vi "Lab Environment Query.vi"() -> ()   [LabVIEW 2012]
uses:
  <vilib>/Utility/miscctls.llb/LVPointTypeDef.ctl
  <vilib>/addons/database/Auxilliary.llb/DB Tools Cursor Type.ctl
  <userlib>/_OpenG.lib/array/array.llb/Index 1D Array Elements (String)__ogtk.vi
  <vilib>/addons/database/Connection.llb/Conn Execute.vi
  <vilib>/addons/database/Recordset.llb/Rec Fetch Recordset Data (R).vi
  <vilib>/addons/database/Recordset.llb/Rec Destroy - Connection.vi
  <vilib>/Utility/file.llb/Write To Spreadsheet File (string).vi
  <vilib>/addons/database/_DB Variant To Data/Database Variant To Data.xnode
  <vilib>/addons/database/NI_Database_API.lvlib
panel:
  in  "stop":bool
  in  "Tab Control":T1(tab)
  in  "Active Y Scale":u16(ring) items=["Temperature (F)", "Pressure (torr)"]
  in  "X Maximum":dbl format="%<%I:%M:%S %p\n%m/%d/%Y>T"
  in  "X Autoscale":bool=TRUE
  in  "X Minimum":dbl format="%<%I:%M:%S %p\n%m/%d/%Y>T"
  in  "Y Autoscale":bool=TRUE
  in  "Y Maximum":dbl
  in  "Y Minimum":dbl
  in  "Plot":bool
  in  "Limits":T2
  in  "Lab Properties":i32[](listbox)
  out "XY Graph":cluster{ext[], dbl[]}[](graph)
  in  "Write":bool
  in  "Pull Data":bool
  in  "Limits 2":T2
  out "Lab Environment Data":string[][](table)
  in  "Save Path":path=path "C:/Users/Clavius/Desktop/Database Query files/New_Pelletron_Query.csv"
  out "error out":errorcluster
  in  "Clear Errors?":bool
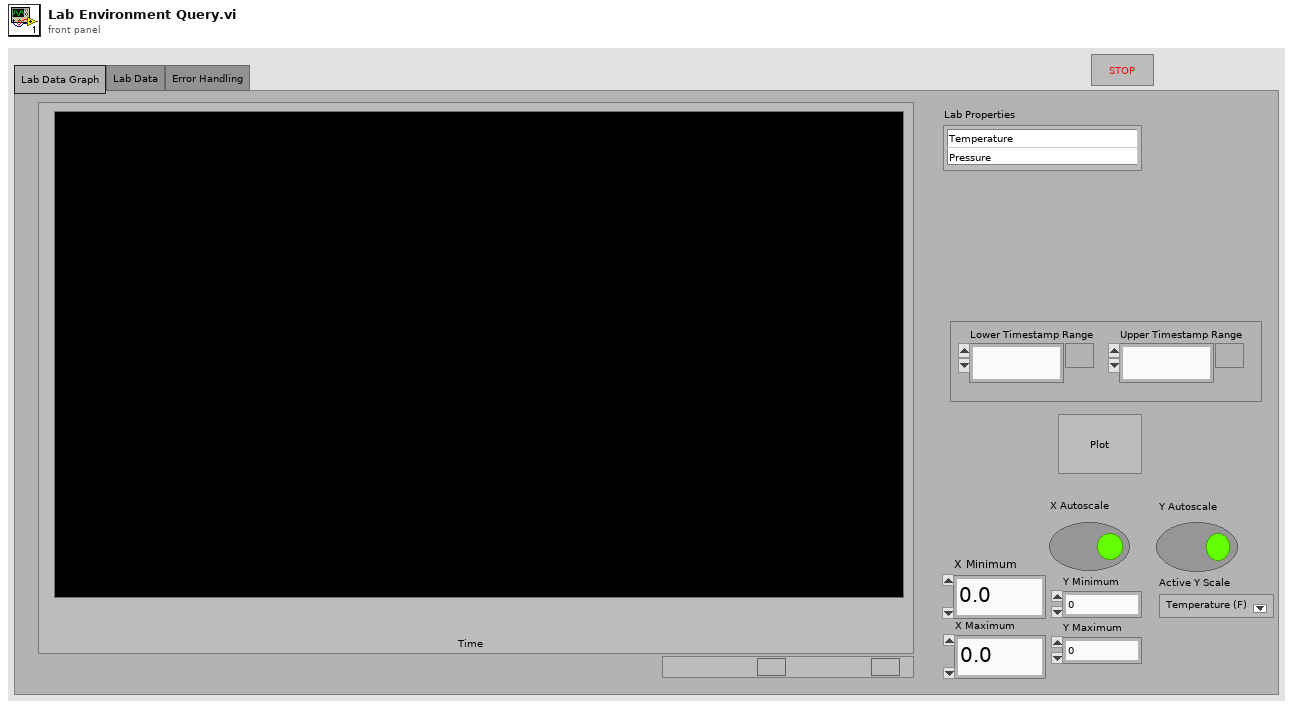
[diagram p1: front panel]
types:
  T1 = enum32{"Lab Data Graph", "Lab Data", "Error Handling"}
  T2 = cluster{"Lower Timestamp Range":timestamp, "Upper Timestamp Range":timestamp}
  T3 = typedef "LVPointTypeDef.ctl" = cluster{"Horizontal":i16, "Vertical":i16}
  T4 = typedef "NI_Database_API.lvlib/DB Tools Cursor Type.ctl" = enum16{"forward-only", "keyset", "dynamic", "static"}
  T5 = cluster{"Integer Timestamp":dbl[], "Temperature (F)":dbl[], "Pressure (torr)":dbl[]}
  T6 = typedef "NI_Database_API.lvlib/Conn ObjectReference.ctl" = refnum<k1>
  T7 = typedef "NI_Database_API.lvlib/Rec ObjectReference.ctl" = refnum<k1>
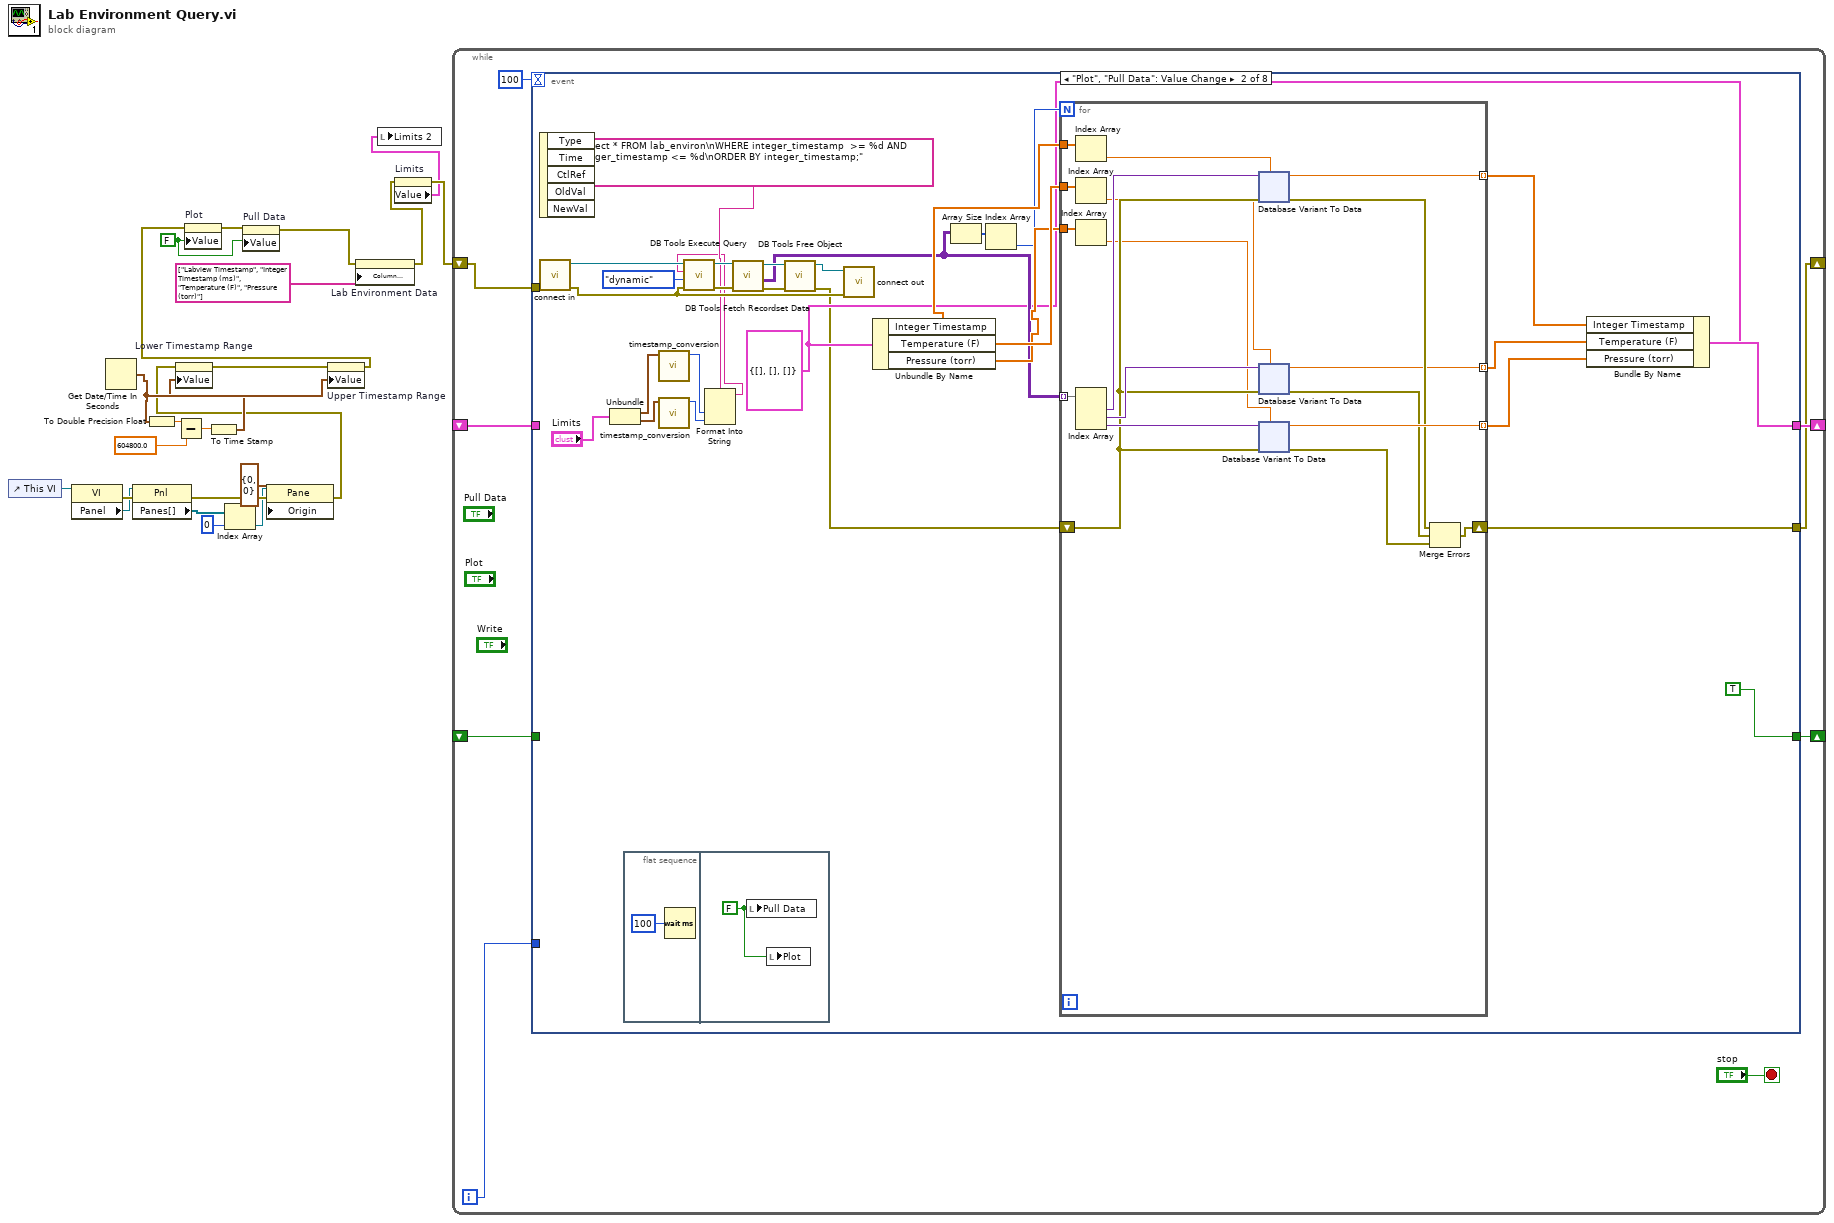
[diagram p0: block diagram]
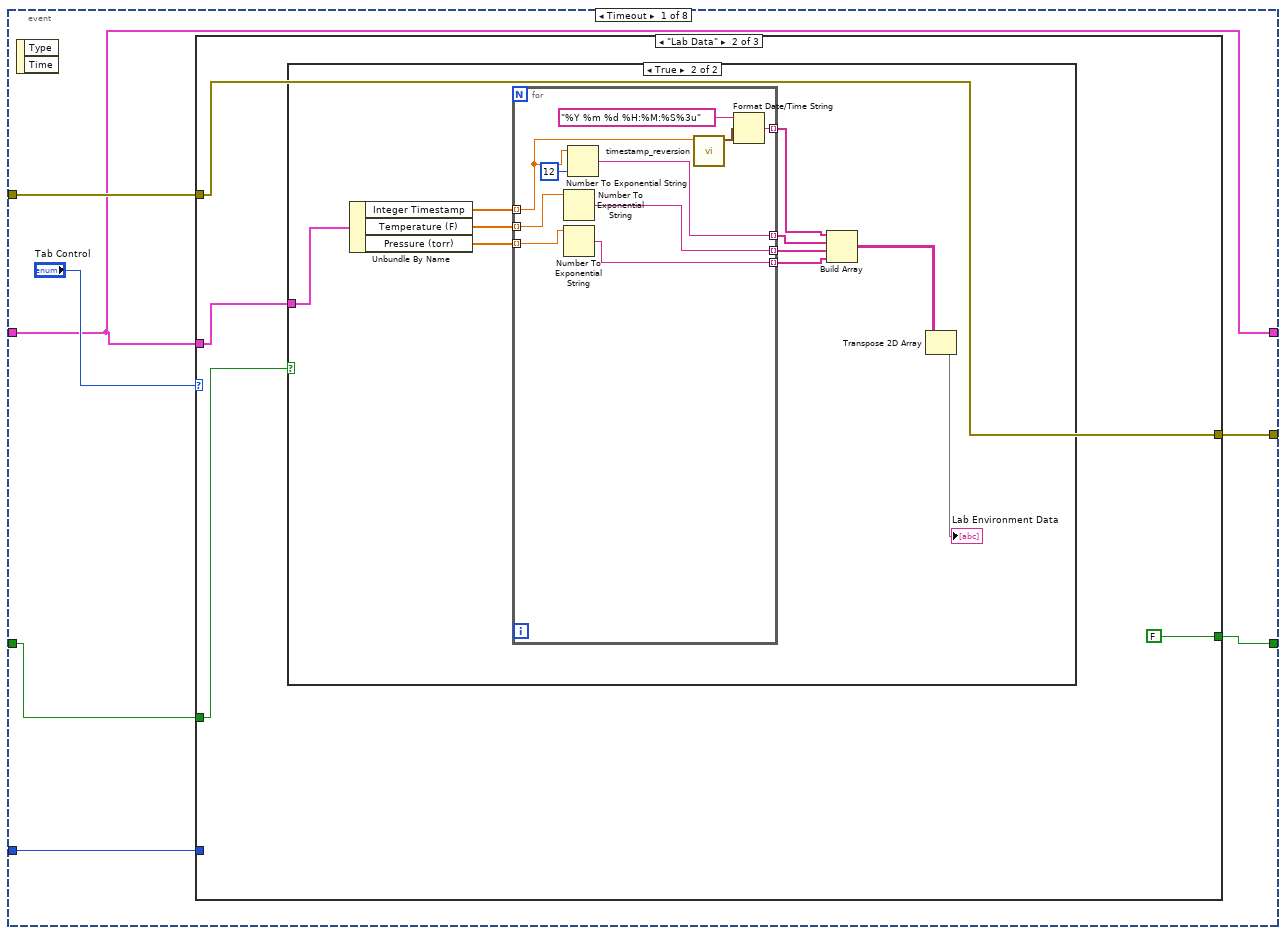
[diagram p2: hidden frame]
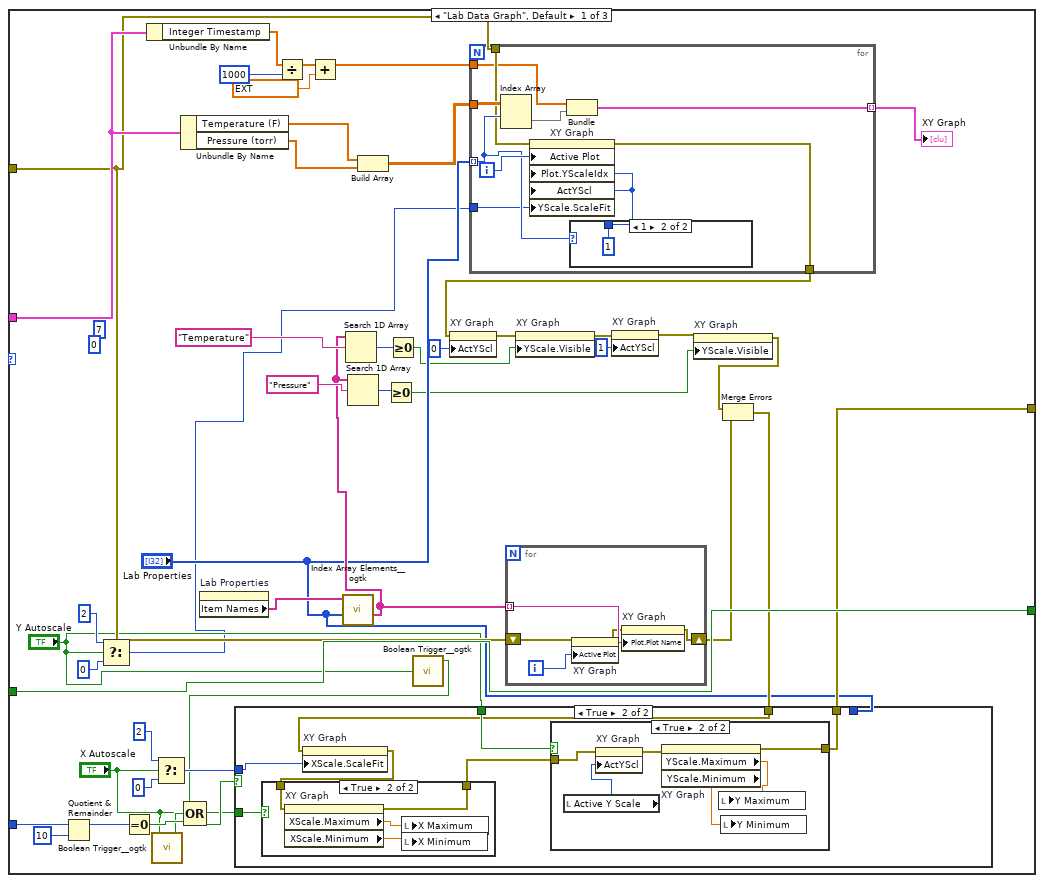
[diagram p3: hidden frame]
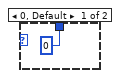
[diagram p7: hidden frame]
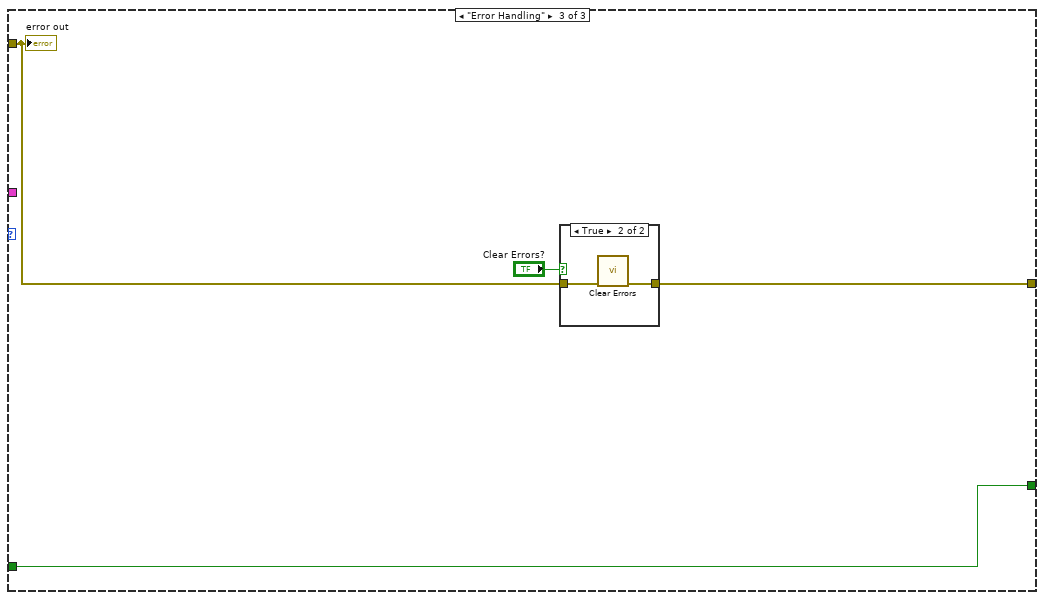
[diagram p9: hidden frame]
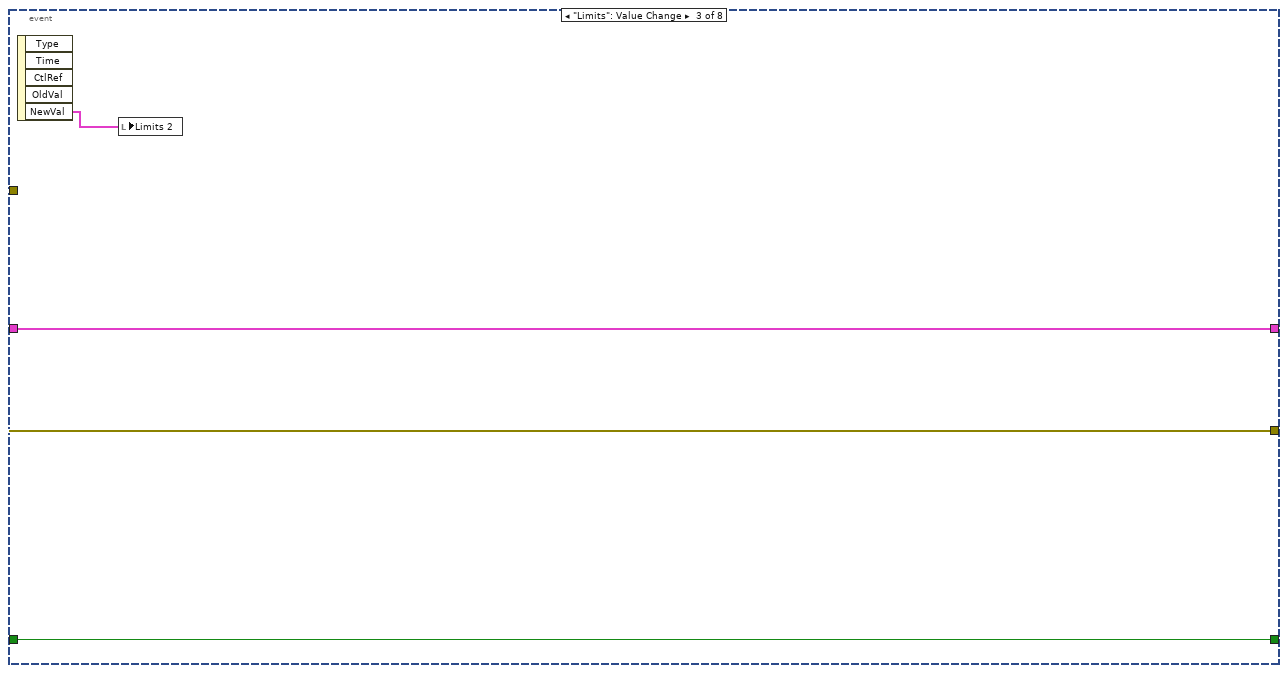
[diagram p11: hidden frame]
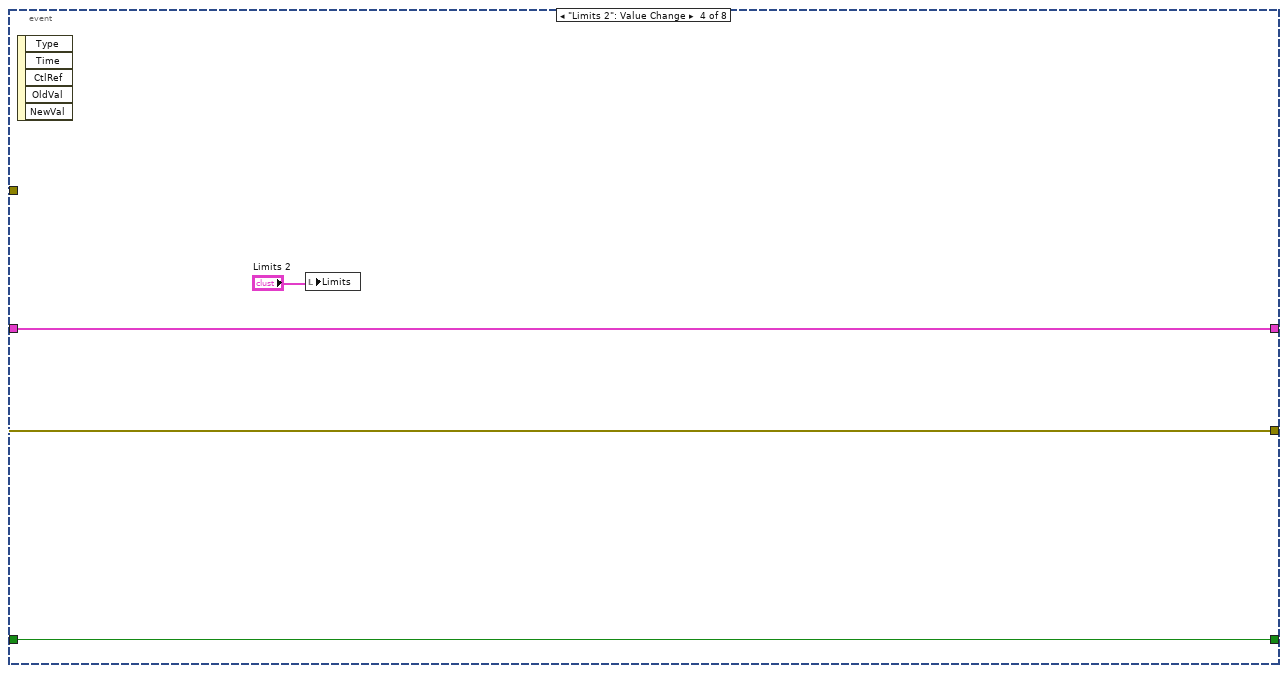
[diagram p12: hidden frame]
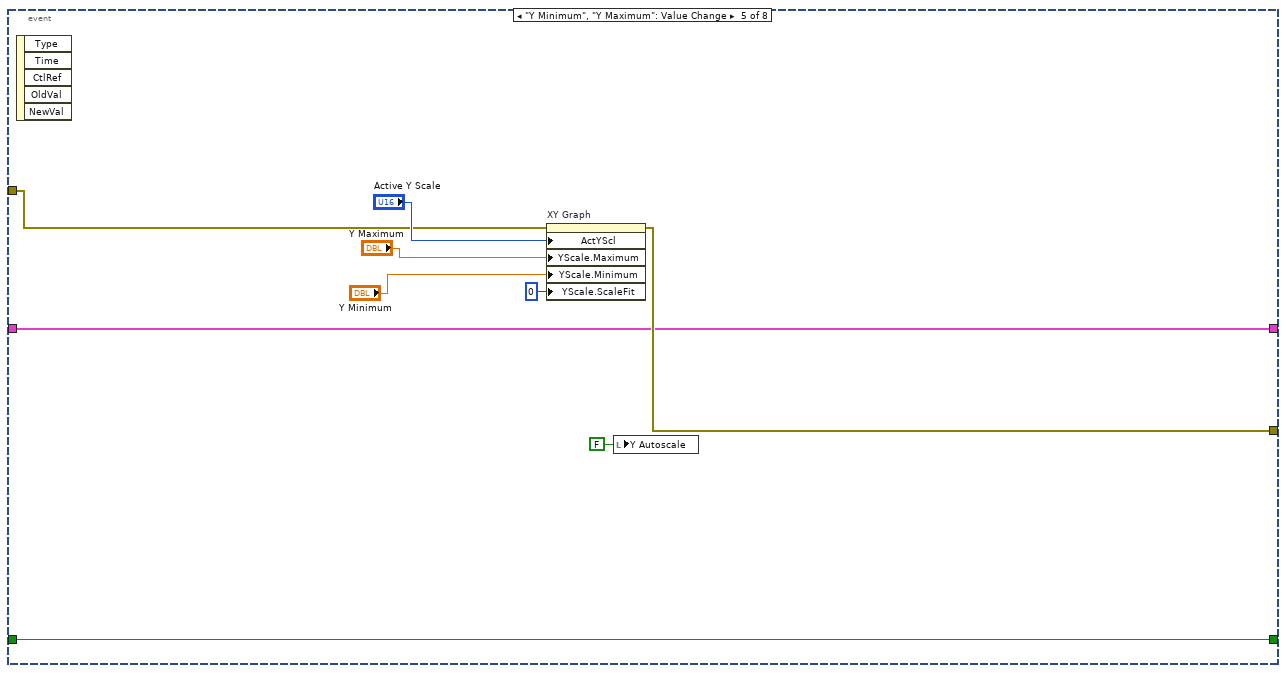
[diagram p13: hidden frame]
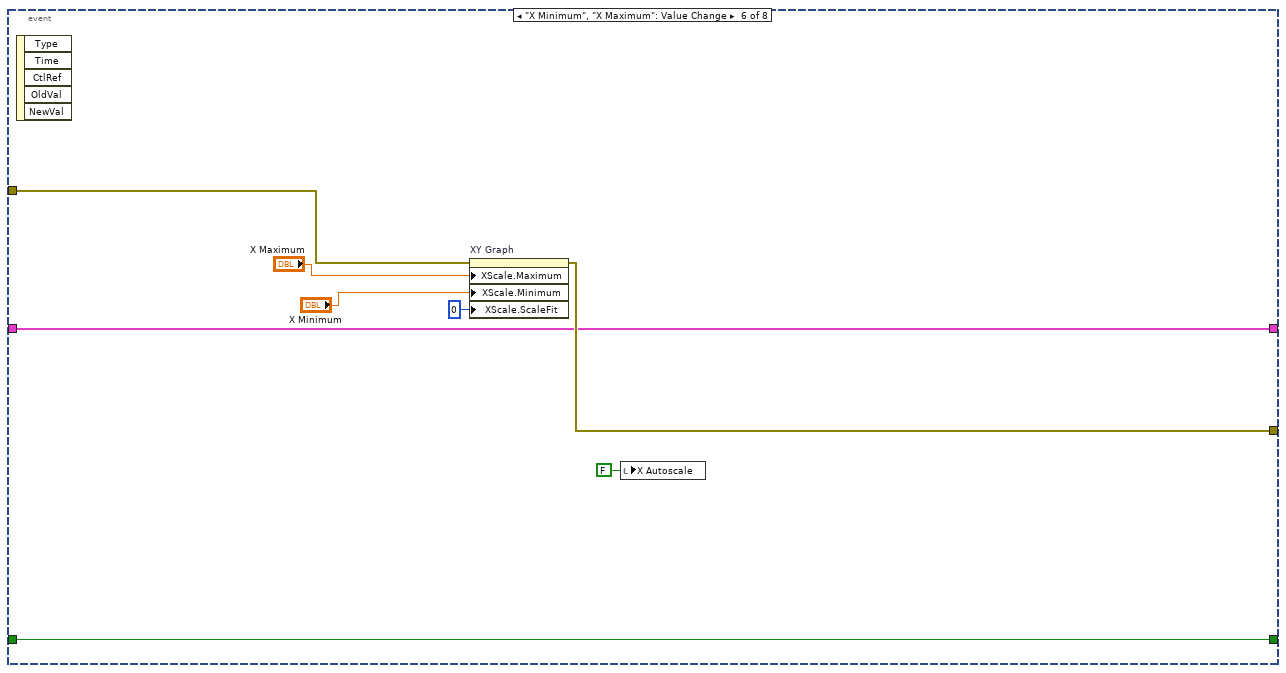
[diagram p14: hidden frame]
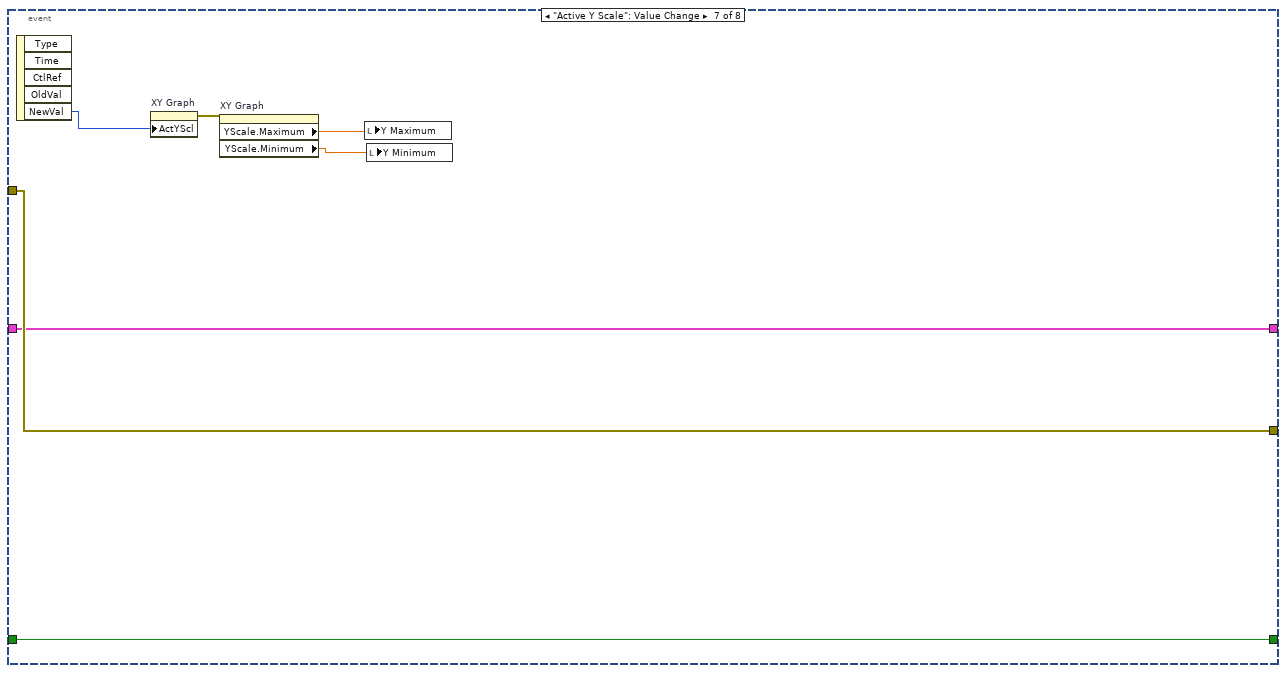
[diagram p15: hidden frame]
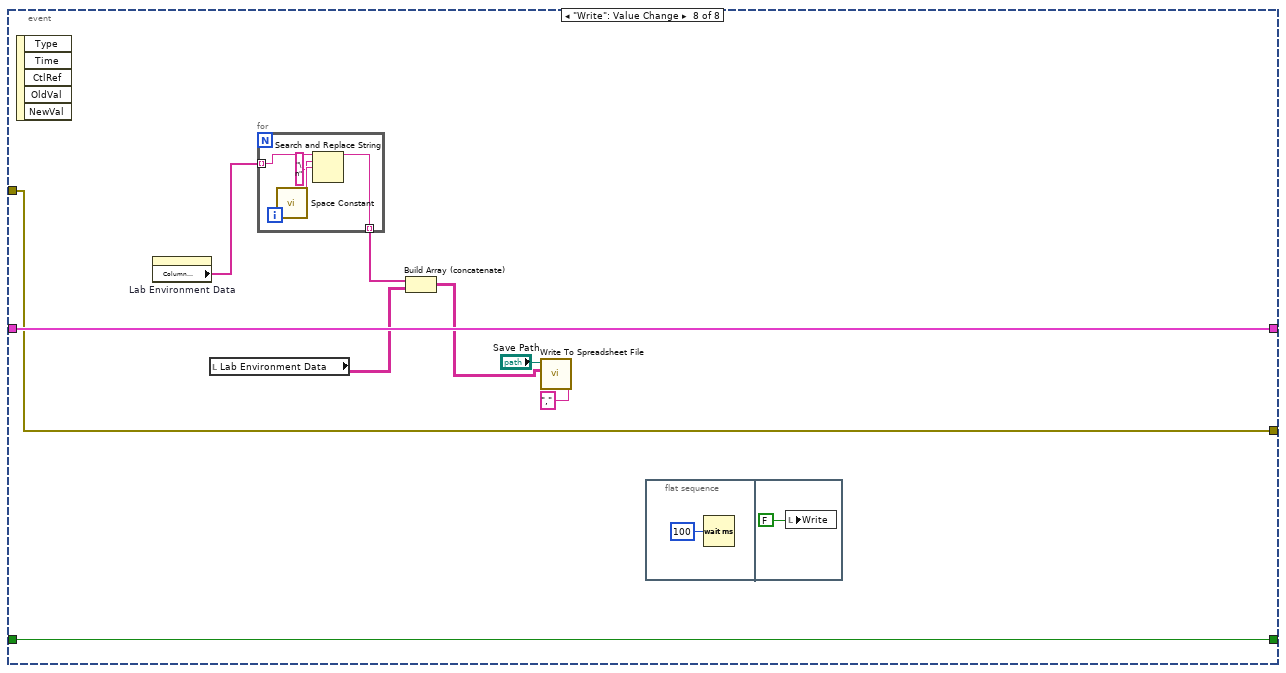
[diagram p16: hidden frame]
diagram:
  w20 = FALSE ("Plot")
  n1 = control-ref of="This VI"() -> (w9:refnum<vi>)
  n2 = property class="VI"(reference=w9) -> (error out=w8:errorcluster, "Panel"=w7:refnum<vi>)  [unwired: 1 in, 1 out]
  n3 = Get Date/Time In Seconds() -> (seconds since 1Jan1904=w17:timestamp)
  n4 = property class="Pnl"(reference=w7, error in=w8) -> (error out=w6:errorcluster, "Panes[]"=w5:refnum<vi>[])  [unwired: 1 out]
  n5 = To Double Precision Float(number=w17) -> (double precision float=w16:dbl)
  n6 = Subtract(x=w16, y=604800.0) -> (x-y=w14:dbl)
  n7 = To Time Stamp(1:w14) -> (0:w13:timestamp)
  n8 = Index Array(array=w5, index=0) -> (element=w3:refnum<vi>)
  n9 = property class="Pane"(reference=w3, error in=w6, "Origin"=T3 {"Horizontal"=0, "Vertical"=0}) -> (error out=w1:errorcluster)  [unwired: 1 out]
  n10 = property on="Lower Timestamp Range" class="AbsTime (strict)"(error in=w1, "Value"=w13) -> (error out=w19:errorcluster)  [unwired: 1 in, 1 out]
  n11 = property on="Upper Timestamp Range" class="AbsTime (strict)"(error in=w19, "Value"=w17) -> (error out=w18:errorcluster)  [unwired: 1 in, 1 out]
  n12 = property on="Plot" class="Bool (strict)"(error in=w18, "Value"=w20) -> (error out=w22:errorcluster)  [unwired: 1 in, 1 out]
  n13 = property on="Pull Data" class="Bool (strict)"(error in=w22, "Value"=w20) -> (error out=w21:errorcluster)  [unwired: 1 in, 1 out]
  n14 = property on="Lab Environment Data" class="Tbl (strict)"(error in=w21, "Column Headers[]"=string[] ["Labview Timestamp", "Integer Timestamp (ms)", "Temperature (F)", "Pressure (torr)"]) -> (error out=w12:errorcluster)  [unwired: 1 in, 1 out]
  n15 = property on="Limits" class="Clust (strict)"(error in=w12) -> (error out=w11:errorcluster, "Value"=w10:T2)  [unwired: 1 in, 1 out]
  n16 = local write "Limits 2"(w10) -> ()
  n17 = while {
    shift-right: [w29] -> _
    shift-left: w11 -> [w31]
    shift-right: [w30] -> _
    shift-left: _ -> [w28]
    shift-right: [w26] -> _
    shift-left: _ -> [w25]
    i -> [w24]
    stop <- "stop" stop-if-true
    n18 = event shown="[1] \"Plot\", \"Pull Data\": Value Change" {
      selector: _ -> [_ _ _ _ _ _ _ _]
      dyn-events: _ -> [_ _ _ _ _ _ _ _]
      timeout: 100 -> [_ _ _ _ _ _ _ _]
      tunnel: w31 -> [w38 w181 w303 w307 w311 w321 w331 w337]
      tunnel: w28 -> [w36 _ w302 w306 w309 w319 w330 w338]
      tunnel: [w36 w165 w302 w306 w309 w319 w330 w338] -> w30
      tunnel: [w37 w155 w303 w307 w310 w320 w331 w337] -> w29
      tunnel: [w35 TRUE w301 w305 w308 w318 w329 w336] -> w26
      tunnel: w25 -> [w34 _ w301 w305 w308 w318 w329 w336]
      tunnel: w24 -> [w33 _ _ _ _ _ _ _]
      event Timeout {
        n19 = event-data() -> ()  [unwired: 1 in, 2 out]
        n20 = case shown="\"Lab Data\"" "Tab Control" {
          tunnel: w38 -> [w64 w125 w150]
          tunnel: [w62 w125 w149] -> w37
          tunnel: w36 -> [w85 w126 _]
          tunnel: [w84 FALSE w147] -> w35
          tunnel: w34 -> [w84 w123 w147]
          tunnel: w33 -> [w61 _ _]
          frame "Lab Data Graph", Default {
            (unwired) u8 7 ("X Scale.Display Format:Format")
            (unwired) u8 0 ("X Scale.Display Format:Format")
            n21 = Quotient & Remainder(x=w61, y=10) -> (x-y*floor(x/y)=w58:i32)  [unwired: 1 out]
            n22 = Select(t=u8 2 ("X Scale.Scale Fit"), s="Y Autoscale", f=u8 0 ("X Scale.Scale Fit")) -> (s? t:f=w50:u8)
            n23 = Equal To 0?(x=w58) -> (x = 0?=w57:bool)
            n24 = Unbundle By Name(w85) -> ("Integer Timestamp"=w43:dbl[])
            n25 = call <userlib>:"Boolean Trigger__ogtk.vi"("Boolean Input"="X Autoscale") -> ("Rising Edge"=w55:bool)  [unwired: 1 in, 1 out]
            n26 = Select(t=u8 2 ("X Scale.Scale Fit"), s="X Autoscale", f=u8 0 ("X Scale.Scale Fit")) -> (s? t:f=w67:u8)
            n27 = Unbundle By Name(w85) -> ("Temperature (F)"=w83:dbl[], "Pressure (torr)"=w49:dbl[])
            n28 = property on="Lab Properties" class="LstBox (strict)"() -> ("Item Names"=w80:string[])  [unwired: 2 in, 2 out]
            n29 = Divide(x=w43, y=1000 ("Numeric")) -> (x/y=w44:dbl[])
            n30 = Add(x=w44, y=ext 2082844800.0) -> (x+y=w41:ext[])
            n31 = call-poly <userlib>:"Index Array Elements__ogtk.vi"("indices"="Lab Properties", "array"=w80) -> ("elements"=w69:string[])  [unwired: 9 in]
            n32 = Search 1D Array(1D array=w69, element="Temperature") -> (index of element=w76:i32)  [unwired: 1 in]
            n33 = Search 1D Array(1D array=w69, element="Pressure") -> (index of element=w75:i32)  [unwired: 1 in]
            n34 = Build Array(w83, w49) -> (w82:dbl[][])
            n35 = Greater Or Equal To 0?(x=w75) -> (x >= 0?=w46:bool)
            n36 = Greater Or Equal To 0?(x=w76) -> (x >= 0?=w45:bool)
            n37 = call <userlib>:"Boolean Trigger__ogtk.vi"("Boolean Input"="Y Autoscale") -> ("Rising Edge"=w52:bool)  [unwired: 1 in, 1 out]
            n38 = Compound Arithmetic op=OR(w52, w55, w57) -> (w56:bool)
            n39 = for {
              tunnel: "Lab Properties" -> [w116] mode=indexing
              tunnel: w82 -> [w120]
              tunnel: w41 -> [w111]
              tunnel: [w118] -> w81 mode=indexing
              tunnel: w64 -> [w115]
              tunnel: [w114] -> w48
              tunnel: w50 -> [w112]
              i -> [w117]
              n40 = Index Array(array=w120, index (row)=w116) -> (element=w119:dbl[])  [unwired: 1 in]
              n41 = Bundle(w111, w119) -> (w118:cluster{ext[], dbl[]})  [unwired: 1 in]
              n42 = case shown="1" w116 {
                tunnel: [u32 0 ("Plot.Y Scale Index") u32 1 ("Plot.Y Scale Index")] -> w113
                frame 0, Default {
                }
                frame 1 {
                }
              }
              n43 = property on="XY Graph" class="XYGraph (strict)"(error in=w115, "Active Plot"=w117, "Plot.YScaleIdx"=w113, "ActYScl"=w113, "YScale.ScaleFit"=w112) -> (error out=w114:errorcluster)  [unwired: 1 in, 1 out]
            }
            "XY Graph" <- w81
            n44 = property on="XY Graph" class="XYGraph (strict)"(error in=w48, "ActYScl"=0 ("Active Y Scale")) -> (error out=w73:errorcluster)  [unwired: 1 in, 1 out]
            n45 = for {
              tunnel: w69 -> [w109] mode=indexing
              shift-right: [w107] -> w79
              shift-left: w64 -> [w106]
              i -> [w110]
              n46 = property on="XY Graph" class="XYGraph (strict)"(error in=w106, "Active Plot"=w110) -> (error out=w108:errorcluster)  [unwired: 1 in, 1 out]
              n47 = property on="XY Graph" class="XYGraph (strict)"(error in=w108, "Plot.Plot Name"=w109) -> (error out=w107:errorcluster)  [unwired: 1 in, 1 out]
            }
            n48 = property on="XY Graph" class="XYGraph (strict)"(error in=w73, "YScale.Visible"=w45) -> (error out=w72:errorcluster)  [unwired: 1 in, 1 out]
            n49 = property on="XY Graph" class="XYGraph (strict)"(error in=w72, "ActYScl"=1 ("Active Y Scale")) -> (error out=w70:errorcluster)  [unwired: 1 in, 1 out]
            n50 = property on="XY Graph" class="XYGraph (strict)"(error in=w70, "YScale.Visible"=w46) -> (error out=w47:errorcluster)  [unwired: 1 in, 1 out]
            n51 = Merge Errors(w47, w79) -> (w63:errorcluster)
            n52 = case shown="True" w56 {
              tunnel: w67 -> [_ w93]
              tunnel: "Y Autoscale" -> [_ w92]
              tunnel: w63 -> [w86 w89]
              tunnel: [w86 w87] -> w62
              tunnel: "X Autoscale" -> [_ w88]
              tunnel: "Lab Properties" -> [_ _]
              frame False {
              }
              frame True {
                n53 = property on="XY Graph" class="XYGraph (strict)"(error in=w89, "XScale.ScaleFit"=w93) -> (error out=w91:errorcluster)  [unwired: 1 in, 1 out]
                n54 = case shown="True" w88 {
                  tunnel: w91 -> [w101 w103]
                  tunnel: [w101 w102] -> w90
                  frame False {
                  }
                  frame True {
                    n55 = property on="XY Graph" class="XYGraph (strict)"(error in=w103) -> (error out=w102:errorcluster, "XScale.Maximum"=w105:dbl, "XScale.Minimum"=w104:dbl)  [unwired: 1 in, 1 out]
                    n56 = local write "X Maximum"(w105) -> ()
                    n57 = local write "X Minimum"(w104) -> ()
                  }
                }
                n58 = case shown="True" w92 {
                  tunnel: w90 -> [w94 w96]
                  tunnel: [w94 w95] -> w87
                  frame False {
                  }
                  frame True {
                    n59 = local read "Active Y Scale"() -> (w99:u16)
                    n60 = property on="XY Graph" class="XYGraph (strict)"(error in=w96, "ActYScl"=w99) -> (error out=w100:errorcluster)  [unwired: 1 in, 1 out]
                    n61 = property on="XY Graph" class="XYGraph (strict)"(error in=w100) -> (error out=w95:errorcluster, "YScale.Maximum"=w98:dbl, "YScale.Minimum"=w97:dbl)  [unwired: 1 in, 1 out]
                    n62 = local write "Y Maximum"(w98) -> ()
                    n63 = local write "Y Minimum"(w97) -> ()
                  }
                }
              }
            }
          }
          frame "Lab Data" {
            n64 = case shown="True" w123 {
              tunnel: w126 -> [_ w136]
              frame False {
              }
              frame True {
                n65 = Unbundle By Name(w136) -> ("Integer Timestamp"=w135:dbl[], "Temperature (F)"=w134:dbl[], "Pressure (torr)"=w133:dbl[])
                n66 = for {
                  tunnel: w135 -> [w139] mode=indexing
                  tunnel: w134 -> [w141] mode=indexing
                  tunnel: w133 -> [w140] mode=indexing
                  tunnel: [w144] -> w128 mode=indexing
                  tunnel: [w143] -> w132 mode=indexing
                  tunnel: [w142] -> w131 mode=indexing
                  tunnel: [w138] -> w127 mode=indexing
                  n67 = Number To Exponential String(number=w141) -> (E-format string=w143:string)  [unwired: 3 in]
                  n68 = Number To Exponential String(number=w140) -> (E-format string=w142:string)  [unwired: 3 in]
                  n69 = Number To Exponential String(number=w139, precision (6)=i16 12) -> (E-format string=w138:string)  [unwired: 2 in]
                  n70 = call "timestamp_reversion.vi"("Integer Timestamp"=w139) -> ("time stamp"=w145:timestamp)  [unwired: 8 in, 1 out]
                  n71 = Format Date/Time String(time format string (%c)="%Y %m %d %H:%M:%S%3u", seconds (now)=w145) -> (date/time string=w144:string)  [unwired: 1 in]
                }
                n72 = Build Array(w128, w127, w132, w131) -> (w130:string[][])
                n73 = Transpose 2D Array(2D array=w130) -> (transposed array=→"Lab Environment Data":string[][])
              }
            }
          }
          frame "Error Handling" {
            n74 = case shown="True" "Clear Errors?" {
              tunnel: w150 -> [w151 w153]
              tunnel: [w151 w152] -> w149
              frame False {
              }
              frame True {
                n75 = call <vilib>:"Clear Errors.vi"("error in (no error)"=w153) -> ("error out"=w152:errorcluster)  [unwired: 6 in]
              }
            }
            "error out" <- w150
          }
        }
      }
      event "Plot", "Pull Data": Value Change {
        w164 = T5 {"Integer Timestamp"=[], "Temperature (F)"=[], "Pressure (torr)"=[]} ("Cluster")
        n76 = event-data() -> ()  [unwired: 1 in, 5 out]
        n77 = call "connect in.vi"("error in (no error)"=w181) -> ("error out"=w178:errorcluster, "Database Connection"=w182:T6)  [unwired: 6 in, 1 out]
        n78 = Unbundle("Limits") -> ("Lower Timestamp Range"=w160:timestamp, "Upper Timestamp Range"=w159:timestamp)
        n79 = flat-sequence {
          frame #0 {
            n80 = Wait (ms)(milliseconds to wait=u32 100) -> ()  [unwired: 1 out]
          }
          frame #1 {
            w185 = FALSE ("Pull Data")
            n81 = local write "Pull Data"(w185) -> ()
            n82 = local write "Plot"(w185) -> ()
          }
        }
        n83 = call "timestamp_conversion.vi"("Time Stamp"=w160) -> ("Integer Time"=w158:i64)  [unwired: 8 in, 1 out]
        n84 = call "timestamp_conversion.vi"("Time Stamp"=w159) -> ("Integer Time"=w157:i64)  [unwired: 8 in, 1 out]
        n85 = Format Into String(format string="Select * FROM lab_environ\nWHERE integer_timestamp  >= %d AND integer_timestamp <= %d\nORDER BY integer_timestamp;", w158, w157) -> (resulting string=w162:string)  [unwired: 2 in, 1 out]
        n86 = call-poly <vilib>:"DB Tools Execute Query.vi"("error in (no error)"=w178, "cursor type"=DB_Tools_Cursor_Type."dynamic", "SQL query"=w162, "connection reference"=w182) -> ("error out"=w179:errorcluster, "recordset reference"=w177:T7)  [unwired: 4 in]
        n87 = call-poly <vilib>:"DB Tools Fetch Recordset Data.vi"("error in (no error)"=w179, "recordset reference"=w177) -> ("error out"=w180:errorcluster, "recordset data"=w171:variant[][], "recordset reference out"=w176:T7)  [unwired: 3 in]
        n88 = call-poly <vilib>:"DB Tools Free Object.vi"("error in (no error)"=w180, "recordset reference"=w176) -> ("error out"=w156:errorcluster, "connection reference"=w175:T6)  [unwired: 8 in]
        n89 = call "connect out.vi"("error in (no error)"=w178, "connection reference"=w175) -> ()  [unwired: 9 in, 1 out]
        n90 = Unbundle By Name(w164) -> ("Integer Timestamp"=w174:dbl[], "Temperature (F)"=w173:dbl[], "Pressure (torr)"=w172:dbl[])
        n91 = Array Size(array=w171) -> (size(s)=w170:i32[])
        n92 = Index Array(array=w170) -> (element=w169:i32)  [unwired: 1 in]
        n93 = for {
          N: w169 -> [_]
          tunnel: w171 -> [w203] mode=indexing
          tunnel: w174 -> [w199]
          tunnel: w173 -> [w198]
          tunnel: w172 -> [w197]
          tunnel: [w186] -> w168 mode=indexing
          tunnel: [w188] -> w167 mode=indexing
          tunnel: [w196] -> w166 mode=indexing
          shift-right: [w192] -> w155
          shift-left: w156 -> [w195]
          n94 = Index Array(array=w199) -> (element=w191:dbl)  [unwired: 1 in]
          n95 = Index Array(array=w198) -> (element=w190:dbl)  [unwired: 1 in]
          n96 = Index Array(array=w197) -> (element=w189:dbl)  [unwired: 1 in]
          n97 = Index Array(array=w203) -> (element #1=w202:variant, element #2=w201:variant, element #3=w200:variant)  [unwired: 3 in]
          n98 = xnode "Database Variant To Data"("database variant"=w202, "error in (no error)"=w195, "type"=w191) -> ("data"=w186:dbl, "error out"=w194:errorcluster)
          n99 = xnode "Database Variant To Data"("database variant"=w201, "error in (no error)"=w195, "type"=w190) -> ("data"=w188:dbl, "error out"=w187:errorcluster)
          n100 = xnode "Database Variant To Data"("database variant"=w200, "error in (no error)"=w195, "type"=w189) -> ("data"=w196:dbl, "error out"=w193:errorcluster)
          n101 = Merge Errors(w194, w187, w193) -> (w192:errorcluster)
        }
        n102 = Bundle By Name(cluster=w164, "Integer Timestamp"=w168, "Temperature (F)"=w167, "Pressure (torr)"=w166) -> (w165:T5)
      }
      event "Limits": Value Change {
        n103 = event-data() -> ("NewVal"=w300:T2)  [unwired: 1 in, 4 out]
        n104 = local write "Limits 2"(w300) -> ()
      }
      event "Limits 2": Value Change {
        n105 = event-data() -> ()  [unwired: 1 in, 5 out]
        n106 = local write "Limits"("Limits 2") -> ()
      }
      event "Y Minimum", "Y Maximum": Value Change {
        n107 = event-data() -> ()  [unwired: 1 in, 5 out]
        n108 = property on="XY Graph" class="XYGraph (strict)"(error in=w311, "ActYScl"="Active Y Scale", "YScale.Maximum"="Y Maximum", "YScale.Minimum"="Y Minimum", "YScale.ScaleFit"=u8 0 ("Y Scale.Scale Fit")) -> (error out=w310:errorcluster)  [unwired: 1 in, 1 out]
        n109 = local write "Y Autoscale"(FALSE ("Y Autoscale")) -> ()
      }
      event "X Minimum", "X Maximum": Value Change {
        n110 = event-data() -> ()  [unwired: 1 in, 5 out]
        n111 = property on="XY Graph" class="XYGraph (strict)"(error in=w321, "XScale.Maximum"="X Maximum", "XScale.Minimum"="X Minimum", "XScale.ScaleFit"=u8 0 ("X Scale.Scale Fit")) -> (error out=w320:errorcluster)  [unwired: 1 in, 1 out]
        n112 = local write "X Autoscale"(FALSE ("X Autoscale")) -> ()
      }
      event "Active Y Scale": Value Change {
        n113 = event-data() -> ("NewVal"=w328:u16)  [unwired: 1 in, 4 out]
        n114 = property on="XY Graph" class="XYGraph (strict)"("ActYScl"=w328) -> (error out=w327:errorcluster)  [unwired: 2 in, 1 out]
        n115 = property on="XY Graph" class="XYGraph (strict)"(error in=w327) -> ("YScale.Maximum"=w326:dbl, "YScale.Minimum"=w325:dbl)  [unwired: 1 in, 2 out]
        n116 = local write "Y Maximum"(w326) -> ()
        n117 = local write "Y Minimum"(w325) -> ()
      }
      event "Write": Value Change {
        n118 = event-data() -> ()  [unwired: 1 in, 5 out]
        n119 = property on="Lab Environment Data" class="Tbl (strict)"() -> ("Column Headers[]"=w335:string[])  [unwired: 2 in, 2 out]
        n120 = local read "Lab Environment Data"() -> (w333:string[][])
        n121 = for {
          tunnel: w335 -> [w344] mode=indexing
          tunnel: [w342] -> w334 mode=indexing
          n122 = call <vilib>:"Space Constant.vi"() -> ("String"=w343:string)
          n123 = Search and Replace String(input string=w344, search string="\n", replace string=w343) -> (result string=w342:string)  [unwired: 5 in, 3 out]
        }
        n124 = Build Array (concatenate)(w334, w333) -> (w332:string[][])
        n125 = call-poly <vilib>:"Write To Spreadsheet File.vi"("delimiter (\\t)"="," ("delimiter (\\t)"), "2D data"=w332, "file path (dialog if empty)"="Save Path") -> ()  [unwired: 5 in, 1 out]
        n126 = flat-sequence {
          frame #0 {
            n127 = Wait (ms)(milliseconds to wait=u32 100) -> ()  [unwired: 1 out]
          }
          frame #1 {
            n128 = local write "Write"(FALSE ("Write")) -> ()
          }
        }
      }
    }
  }
